vi "Subtask1B.vi"() -> ()   [LabVIEW 2016, in "Team234_Project5.lvrbt"]
uses:
  Team234_Project5.lvrbt
  <vilib>/NXT/Subs/LVHSConnector.ctl
  <vilib>/NXT/LegoClasses/BrickReference/BrickReference.lvclass
  <vilib>/NXT/Block Support/NXT_OutputPort.ctl
  <vilib>/NXT/NXTIO Xnodes/NXTIONodeSubVIs/NXTMoveMotors.vi
  <vilib>/NXT/Dual Mode Library/Waits/Wait_Num.vi
  <vilib>/NXT/NXTIO Xnodes/NXTIONodeSubVIs/NXTStopMotors.vi
  <vilib>/NXT/NXTIO Xnodes/NXTIOXNode/NXTIO.xnode
panel:
  in  "Time (1 sec) 7":sgl=1.0
  in  "Time (1 sec) 6":sgl=1.0
  in  "Time (1 sec) 5":sgl=1.0
  in  "Phase 4 - B":i8=75
  in  "Large Motor B Phase 3 and 4":i8=75
  in  "Large Motor A Phase 3 and 4":i8=75
  in  "Loop Executions":i32
  in  "Large Motor B Phase 1":i8=75
  in  "Port Large Motor B":T1=7 items=["Port A", "Port B", "Port C", "Port D"]
  in  "NXT/EV3 2":T2
  in  "Port Large Motor A":T1=7 items=["Port A", "Port B", "Port C", "Port D"]
  in  "NXT/EV3 6":T2
  in  "Large Motor A":i8=75
  in  "Large Motor A Phase 2":i8=75
  in  "Large Motor B Phase 2":i8=75
  in  "Time (1 sec) 3":sgl=1.0
  # "Time of Execution"
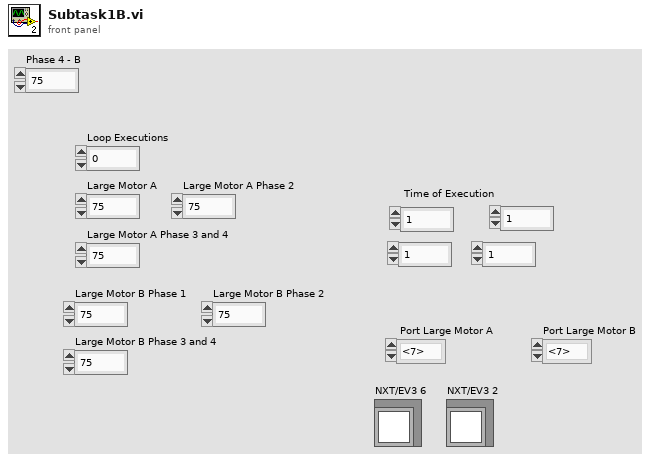
[diagram p1: front panel]
types:
  T1 = typedef "NXT_OutputPort.ctl" = u8
  T2 = typedef "LVHSConnector.ctl" = refnum<class "BrickReference.lvclass">
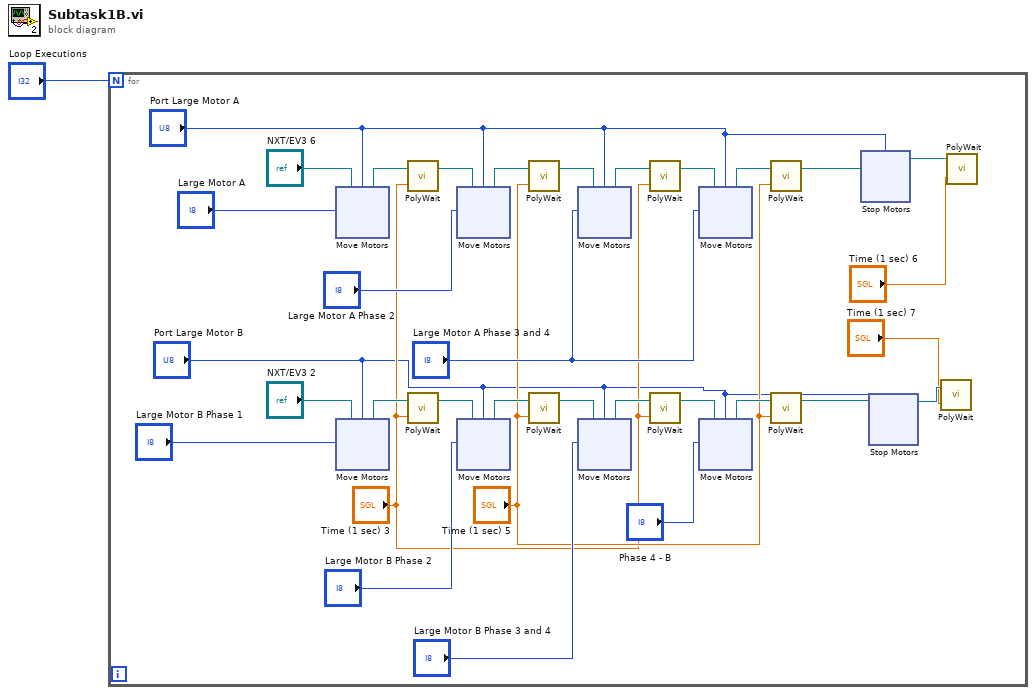
[diagram p0: block diagram]
diagram:
  n1 = for {
    N: "Loop Executions" -> [_]
    n2 = xnode "Move Motors"("Power/Speed 1"="Large Motor A", "Motors"="Port Large Motor A", "NXT/EV3"="NXT/EV3 6") -> ("NXT/EV3"=w31:T2)
    n3 = xnode "Move Motors"("Power/Speed 1"="Large Motor B Phase 1", "Motors"="Port Large Motor B", "NXT/EV3"="NXT/EV3 2") -> ("NXT/EV3"=w27:T2)
    n4 = call-poly <vilib>:"PolyWait.vi"("Time (1 sec)"="Time (1 sec) 3", "NXT/EV3"=w31) -> ("NXT/EV3"=w30:T2)  [unwired: 2 in]
    n5 = call-poly <vilib>:"PolyWait.vi"("Time (1 sec)"="Time (1 sec) 3", "NXT/EV3"=w27) -> ("NXT/EV3"=w26:T2)  [unwired: 2 in]
    n6 = xnode "Move Motors"("Power/Speed 1"="Large Motor A Phase 2", "Motors"="Port Large Motor A", "NXT/EV3"=w30) -> ("NXT/EV3"=w25:T2)
    n7 = xnode "Move Motors"("Power/Speed 1"="Large Motor B Phase 2", "Motors"="Port Large Motor B", "NXT/EV3"=w26) -> ("NXT/EV3"=w24:T2)
    n8 = call-poly <vilib>:"PolyWait.vi"("Time (1 sec)"="Time (1 sec) 5", "NXT/EV3"=w25) -> ("NXT/EV3"=w22:T2)  [unwired: 2 in]
    n9 = call-poly <vilib>:"PolyWait.vi"("Time (1 sec)"="Time (1 sec) 5", "NXT/EV3"=w24) -> ("NXT/EV3"=w20:T2)  [unwired: 2 in]
    n10 = xnode "Move Motors"("Power/Speed 1"="Large Motor A Phase 3 and 4", "Motors"="Port Large Motor A", "NXT/EV3"=w22) -> ("NXT/EV3"=w21:T2)
    n11 = xnode "Move Motors"("Power/Speed 1"="Large Motor B Phase 3 and 4", "Motors"="Port Large Motor B", "NXT/EV3"=w20) -> ("NXT/EV3"=w19:T2)
    n12 = call-poly <vilib>:"PolyWait.vi"("Time (1 sec)"="Time (1 sec) 3", "NXT/EV3"=w21) -> ("NXT/EV3"=w18:T2)  [unwired: 2 in]
    n13 = call-poly <vilib>:"PolyWait.vi"("Time (1 sec)"="Time (1 sec) 3", "NXT/EV3"=w19) -> ("NXT/EV3"=w17:T2)  [unwired: 2 in]
    n14 = xnode "Move Motors"("Power/Speed 1"="Large Motor A Phase 3 and 4", "Motors"="Port Large Motor A", "NXT/EV3"=w18) -> ("NXT/EV3"=w15:T2)
    n15 = xnode "Move Motors"("Power/Speed 1"="Phase 4 - B", "Motors"="Port Large Motor B", "NXT/EV3"=w17) -> ("NXT/EV3"=w16:T2)
    n16 = call-poly <vilib>:"PolyWait.vi"("Time (1 sec)"="Time (1 sec) 5", "NXT/EV3"=w15) -> ("NXT/EV3"=w9:T2)  [unwired: 2 in]
    n17 = call-poly <vilib>:"PolyWait.vi"("Time (1 sec)"="Time (1 sec) 5", "NXT/EV3"=w16) -> ("NXT/EV3"=w5:T2)  [unwired: 2 in]
    n18 = xnode "Stop Motors"("Motors"="Port Large Motor A", "NXT/EV3"=w9) -> ("NXT/EV3"=w7:T2)
    n19 = xnode "Stop Motors"("Motors"="Port Large Motor B", "NXT/EV3"=w5) -> ("NXT/EV3"=w4:T2)
    n20 = call-poly <vilib>:"PolyWait.vi"("Time (1 sec)"="Time (1 sec) 7", "NXT/EV3"=w4) -> ()  [unwired: 2 in, 1 out]
    n21 = call-poly <vilib>:"PolyWait.vi"("Time (1 sec)"="Time (1 sec) 6", "NXT/EV3"=w7) -> ()  [unwired: 2 in, 1 out]
  }
